vi "VerifyToPresentFolderStatus.vi"(11 "Folder Path":path=path "D:/Comics/Marvel") -> (0 "error out":errorcluster, 3 "changed":string[](array[string]))   [LabVIEW 2024]
uses:
  applications/Marvel_API/TypeDefs/comics.reply--cluster.ctl
  applications/Marvel_API/TypeDefs/comic--cluster.ctl
  <vilib>/addons/_JKI.lib/Serialization/JSON/JKI JSON Serialization.lvlib
  <vilib>/addons/_JKI.lib/Serialization/JSON/Deserializer/JSON Deserializer/JSON Deserializer.lvclass
panel:
  out "current series":string
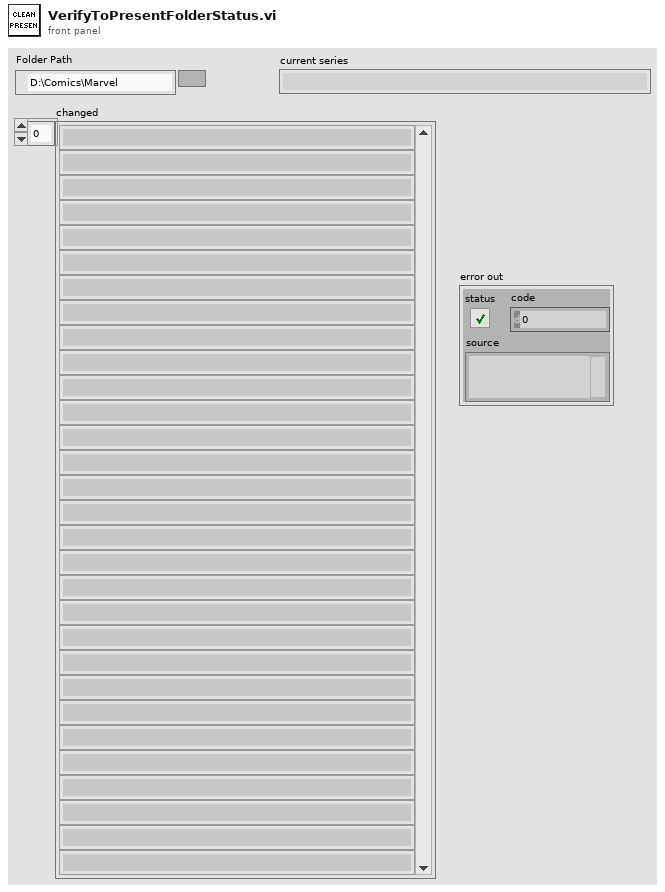
[diagram p1: front panel]
types:
  T1 = typedef "comics.reply--cluster.ctl" = cluster{"code":i32, "status":string, "etag":string, "data":cluster{"offset":i32, "limit":i32, "total":i32, "count":i32, "results":T2[]}}
  T2 = typedef "comic--cluster.ctl" = cluster{"id":i32, "digitalId":i32, "title":string, "issueNumber":i32, "variantDescription":string, "description":string, "modified":variant, "upc":string, "format":string, "pageCount":i32, "resourceURI":string, "urls":cluster{"type":string, "url":string}[], "series":cluster{"resourceURI":string, "name":string}, "dates":cluster{"type":string, "date":string}[], "prices":cluster{"price":dbl, "type":string}[], "thumbnail":cluster{"path":string, "extension":string}, "images":cluster{"path":string, "extension":string}[], "creators":cluster{"available":i32, "returned":i32, "collectionURI":string, "items":cluster{"resourceURI":string, "name":string, "role":string}[]}, "characters":cluster{"available":i32, "returned":i32, "collectionURI":string, "items":cluster{"resourceURI":string, "name":string}[]}, "stories":cluster{"available":i32, "returned":i32, "collectionURI":string, "items":cluster{"resourceURI":string, "name":string, "type":string}[]}, "events":cluster{"available":i32, "returned":i32, "collectionURI":string, "items":cluster{"resourceURI":string, "name":string}[]}}
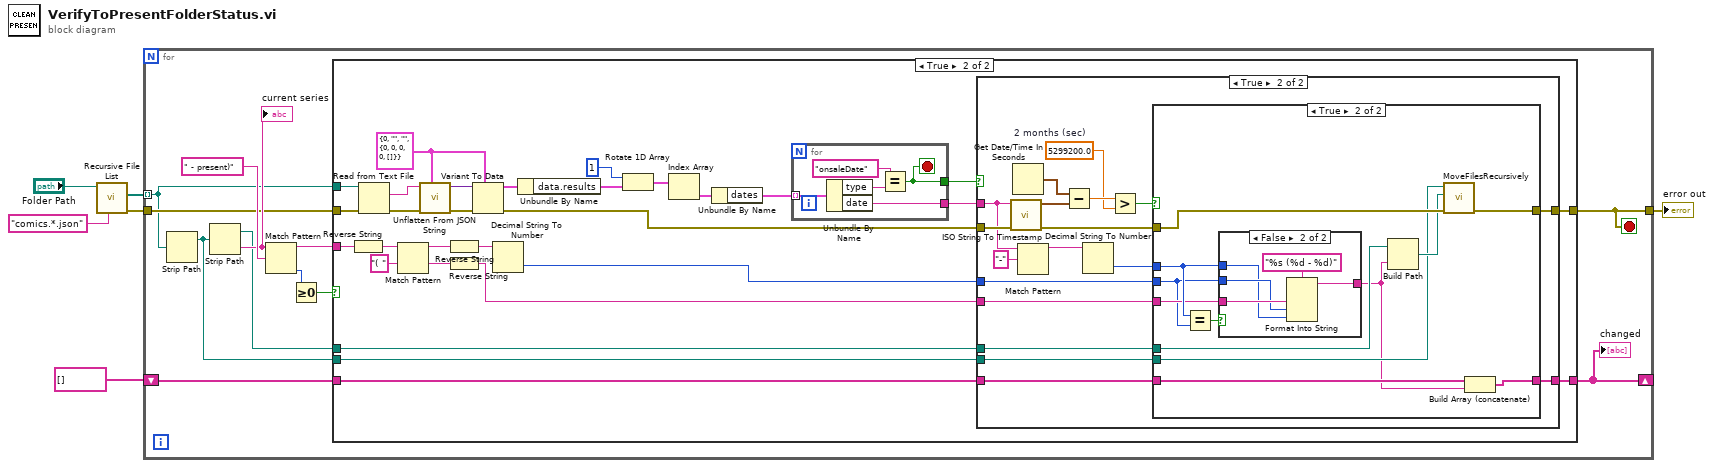
[diagram p0: block diagram]
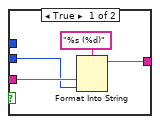
[diagram p5: hidden frame]
diagram:
  n1 = call <vilib>:"Recursive File List.vi"("pattern"="comics.*.json", "Folder Path"="Folder Path") -> ("error out"=w4:errorcluster, "All Files in Dir"=w3:path[])  [unwired: 5 in, 3 out]
  n2 = for {
    tunnel: w4 -> [w14]
    tunnel: w3 -> [w13] mode=indexing
    tunnel: [w9] -> w2
    shift-right: [w7] -> _
    shift-left: string[] [] -> [w8]
    stop <- w9 stop-if-true
    n3 = Strip Path(path=w13) -> (stripped path=w11:path)  [unwired: 1 out]
    n4 = Strip Path(path=w11) -> (stripped path=w10:path, name=w16:string)
    "current series" <- w16
    n5 = Match Pattern(string=w16, regular expression=" - present)") -> (before substring=w12:string, offset past match=w17:i32)  [unwired: 1 in, 2 out]
    n6 = Greater Or Equal To 0?(x=w17) -> (x >= 0?=w15:bool)
    n7 = case shown="True" w15 {
      tunnel: w14 -> [w20 w49]
      tunnel: w13 -> [_ w30]
      tunnel: w12 -> [_ w43]
      tunnel: w11 -> [_ w24]
      tunnel: w10 -> [_ w25]
      tunnel: [w20 w23] -> w9
      tunnel: w8 -> [w19 w22]
      tunnel: [w19 w21] -> w7
      frame False {
      }
      frame True {
        w46 = T1 {"code"=0, "status"="", "etag"="", "data"={"offset"=0, "limit"=0, "total"=0, "count"=0, "results"=[]}} ("reply")
        n8 = Reverse String(1:w43) -> (0:w42:string)
        n9 = Read from Text File(file (use dialog)=w30, error in=w49) -> (text=w47:string, error out=w48:errorcluster)  [unwired: 2 in, 2 out]
        n10 = Match Pattern(string=w42, regular expression="( ") -> (before substring=w29:string, after substring=w27:string)  [unwired: 1 in, 2 out]
        n11 = call <vilib>:"Unflatten From JSON String.vi"("Type and Defaults"=w46, "error in (no error)"=w48, "JSON String"=w47) -> ("error out"=w44:errorcluster, "Variant"=w45:variant)  [unwired: 7 in]
        n12 = Reverse String(1:w29) -> (0:w28:string)
        n13 = Reverse String(1:w27) -> (0:w26:string)
        n14 = Variant To Data(error in=w44, type=w46, Variant=w45) -> (data=w40:T1, error out=w32:errorcluster)
        n15 = Decimal String To Number(string=w28) -> (number=w31:i32)  [unwired: 2 in, 1 out]
        n16 = Unbundle By Name(w40) -> ("data.results"=w39:T2[])
        n17 = Rotate 1D Array(1:w39, 2:1 ("n")) -> (0:w37:T2[])
        n18 = Index Array(array=w37) -> (element=w36:T2)  [unwired: 1 in]
        n19 = Unbundle By Name(w36) -> ("dates"=w35:cluster{"type":string, "date":string}[])
        n20 = for {
          tunnel: w35 -> [w97] mode=indexing
          tunnel: [w94] -> w33
          tunnel: [w93] -> w34
          stop <- w94 stop-if-true
          n21 = Unbundle By Name(w97) -> ("type"=w96:string, "date"=w93:string)
          n22 = Equal?(x="onsaleDate", y=w96) -> (x = y?=w94:bool)
        }
        n23 = case shown="True" w33 {
          tunnel: w34 -> [_ w63]
          tunnel: w32 -> [w51 w69]
          tunnel: w31 -> [_ w59]
          tunnel: w26 -> [_ w58]
          tunnel: w25 -> [_ w56]
          tunnel: w24 -> [_ w55]
          tunnel: [w51 w54] -> w23
          tunnel: w22 -> [w50 w53]
          tunnel: [w50 w52] -> w21
          frame False {
          }
          frame True {
            w65 = 5299200.0  # 2 months (sec)
            n24 = call <vilib>:"ISO String To Timestamp.vi"("error in (no error)"=w69, "ISO Timestamp String"=w63) -> ("error out"=w57:errorcluster, "Time Stamp"=w68:timestamp)  [unwired: 8 in]
            n25 = Get Date/Time In Seconds() -> (seconds since 1Jan1904=w67:timestamp)
            n26 = Match Pattern(string=w63, regular expression="-") -> (before substring=w61:string)  [unwired: 1 in, 3 out]
            n27 = Subtract(x=w67, y=w68) -> (x-y=w66:dbl)
            n28 = Decimal String To Number(string=w61) -> (number=w60:i32)  [unwired: 2 in, 1 out]
            n29 = Greater?(x=w66, y=w65) -> (0:w64:bool)
            n30 = case shown="True" w64 {
              tunnel: w60 -> [_ w82]
              tunnel: w59 -> [_ w80]
              tunnel: w58 -> [_ w81]
              tunnel: w57 -> [w71 w79]
              tunnel: w56 -> [_ w78]
              tunnel: w55 -> [_ w76]
              tunnel: [w71 w75] -> w54
              tunnel: w53 -> [w70 w74]
              tunnel: [w70 w72] -> w52
              frame False {
              }
              frame True {
                n31 = Equal?(x=w82, y=w80) -> (x = y?=w83:bool)
                n32 = case shown="False" w83 {
                  tunnel: w82 -> [_ w88]
                  tunnel: w81 -> [w86 w91]
                  tunnel: w80 -> [w85 w90]
                  tunnel: [w84 w89] -> w73
                  frame True {
                    n33 = Format Into String(format string="%s (%d)", w86, w85) -> (resulting string=w84:string)  [unwired: 2 in, 1 out]
                  }
                  frame False {
                    n34 = Format Into String(format string="%s (%d - %d)", w91, w90, w88) -> (resulting string=w89:string)  [unwired: 2 in, 1 out]
                  }
                }
                n35 = Build Path(base path=w78, name or relative path=w73) -> (appended path=w77:path)
                n36 = call "MoveFilesRecursively.vi"("error in"=w79, "Dest Path"=w77, "Source Path"=w76) -> ("error out"=w75:errorcluster)  [unwired: 8 in]
                n37 = Build Array (concatenate)(w74, w73) -> (w72:string[])
              }
            }
          }
        }
      }
    }
    "changed" <- w7
  }
  "error out" <- w2
